vi "Climbing2.vi"(0 "Start":bool) -> ()   [LabVIEW 2018]
uses:
  <vilib>/Rock Robotics/WPI/Solenoid/WPI_SolenoidValue.ctl
  <vilib>/Rock Robotics/WPI/Utilities/WPI_GetSetVariantRefNum.vi
  Robot Global Data.vi
  <vilib>/Rock Robotics/WPI/Solenoid/WPI_SolenoidSetEnum.vi
  <vilib>/Rock Robotics/WPI/RobotDrive/WPI_RobotDriveArcadeDrive_Standard(NoSaturation).vi
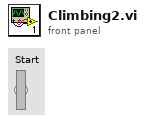
[diagram p1: front panel]
types:
  T1 = typedef "WPI_DigitalInputDevRef.ctl" = cluster{"DevStatus":errorcluster, "DIO Channel":T2}
  T2 = typedef "FPGA_DIOChannel.ctl" = enum8{"DIO 0", "DIO 1", "DIO 2", "DIO 3", "DIO 4", "DIO 5", "DIO 6", "DIO 7", "DIO 8", "DIO 9", "DIO MXP 0", "DIO MXP 1", "DIO MXP 2", "DIO MXP 3", "DIO MXP 4", "DIO MXP 5", "DIO MXP 6", "DIO MXP 7", "DIO MXP 8", "DIO MXP 9", "DIO MXP 10", "DIO MXP 11", "DIO MXP 12", "DIO MXP 13", "DIO MXP 14", "DIO MXP 15", "SPI Port CS1", "SPI Port CS2", "SPI Port CS3", "SPI Port MISO", "SPI Port MOSI", "Invalid"}
  T3 = typedef "WPI_SolenoidDevRef.ctl" = cluster{"DevStatus":errorcluster, "Pneumatics Control Module":u8, "Forward Solenoid Channel":T4, "Reverse Solenoid Channel":T4}
  T4 = typedef "WPI_SolenoidChannel.ctl" = enum8{"Solenoid 0", "Solenoid 1", "Solenoid 2", "Solenoid 3", "Solenoid 4", "Solenoid 5", "Solenoid 6", "Solenoid 7", "Invalid"}
  T5 = typedef "WPI_RobotDriveDevRef.ctl" = cluster{"DevStatus":errorcluster, "Motors[]":T6[], "Square Inputs":bool, "Max Output":dbl}
  T6 = typedef "WPI_MotorControlDeviceRef.ctl" = cluster{"DeviceStatus":errorcluster, "Type":T7, "PWM":cluster{"PWM Channel":T8, "DeadBand":T9}, "CAN":cluster{"Device Number":u8, "SetOutput VI Ref":variant, "GetOutput VI Ref":variant, "Enable VI Ref":variant, "Disable VI Ref":variant, "Data":variant}, "Invert":bool, "DIO PWM":cluster{"PWM \"Enable\" Channel":T8, "DIOChannel":T2, "PWM Rate":dbl}}
  T7 = typedef "WPI_MotorControlType.ctl" = enum16{"PWM", "CAN", "DIO PWM"}
  T8 = typedef "FPGA_DIOPWMChannel.ctl" = enum8{"PWM 0", "PWM 1", "PWM 2", "PWM 3", "PWM 4", "PWM 5", "PWM 6", "PWM 7", "PWM 8", "PWM 9", "PWM MXP 0", "PWM MXP 1", "PWM MXP 2", "PWM MXP 3", "PWM MXP 4", "PWM MXP 5", "PWM MXP 6", "PWM MXP 7", "PWM MXP 8", "PWM MXP 9", "Invalid"}
  T9 = typedef "WPI_PWMDeadband.ctl" = cluster{"Name":string, "maxPositivePwm":i32, "minPositivePwm":i32, "centerPwm":i32, "maxNegativePwm":i32, "minNegativePwm":i32, "angularRange":u16}
  T10 = typedef "WPI_SolenoidValue.ctl" = enum16{"Off", "On", "Forward", "Reverse"}
  T11 = cluster{"X-Axis":dbl, "Y-Axis":dbl, "Z-Axis":dbl}
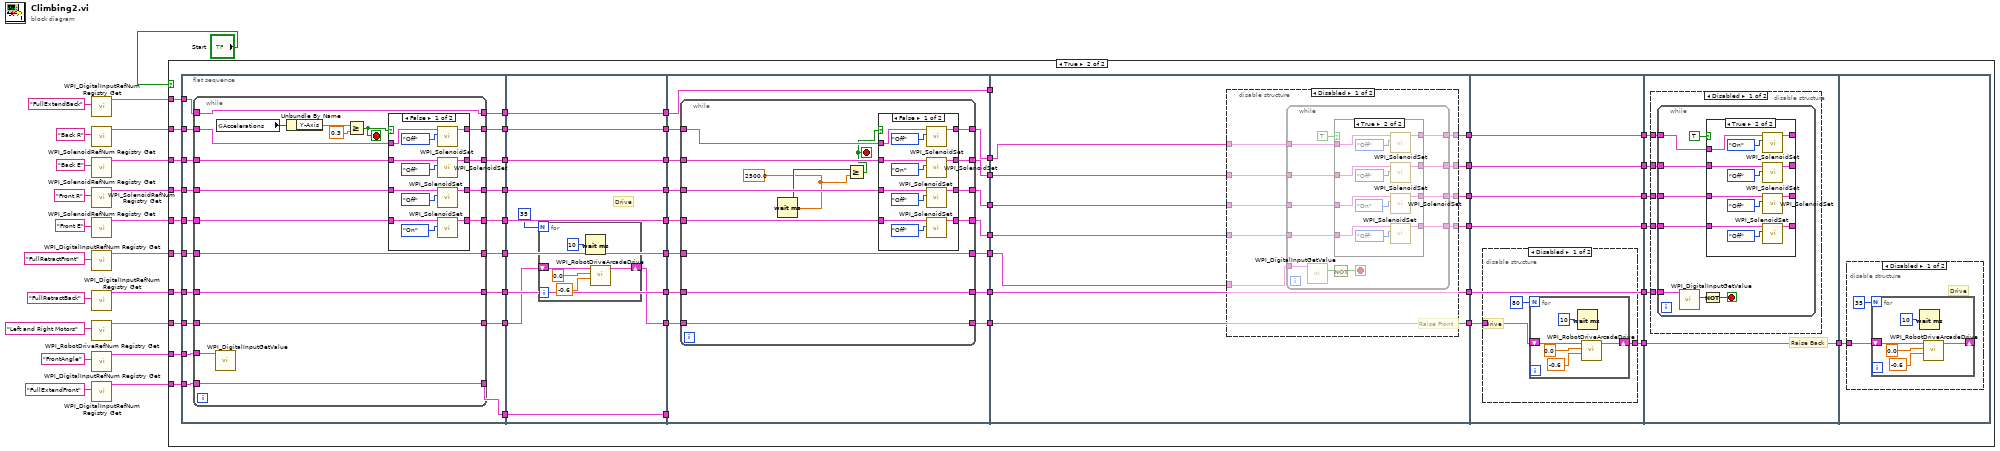
[diagram p0: block diagram]
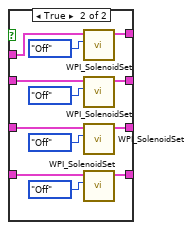
[diagram p3: hidden frame]
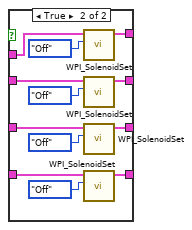
[diagram p4: hidden frame]
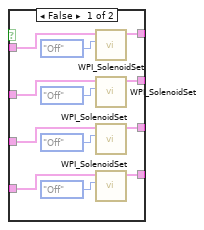
[diagram p5: hidden frame]
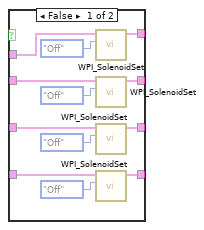
[diagram p8: hidden frame]
diagram:
  n1 = call <vilib>:"WPI_DigitalInputRefNum Registry Get.vi"("refnum name"="FullExtendBack") -> ("DigitalInputDevRef"=w21:T1)  [unwired: 9 in, 1 out]
  n2 = call <vilib>:"WPI_SolenoidRefNum Registry Get.vi"("refnum name"="Back R") -> ("SolenoidDevRef"=w9:T3)  [unwired: 9 in, 1 out]
  n3 = call <vilib>:"WPI_SolenoidRefNum Registry Get.vi"("refnum name"="Back E") -> ("SolenoidDevRef"=w7:T3)  [unwired: 9 in, 1 out]
  n4 = call <vilib>:"WPI_SolenoidRefNum Registry Get.vi"("refnum name"="Front R") -> ("SolenoidDevRef"=w8:T3)  [unwired: 9 in, 1 out]
  n5 = call <vilib>:"WPI_SolenoidRefNum Registry Get.vi"("refnum name"="Front E") -> ("SolenoidDevRef"=w6:T3)  [unwired: 9 in, 1 out]
  n6 = call <vilib>:"WPI_DigitalInputRefNum Registry Get.vi"("refnum name"="FullRetractFront") -> ("DigitalInputDevRef"=w19:T1)  [unwired: 9 in, 1 out]
  n7 = call <vilib>:"WPI_DigitalInputRefNum Registry Get.vi"("refnum name"="FullRetractBack") -> ("DigitalInputDevRef"=w17:T1)  [unwired: 9 in, 1 out]
  n8 = call <vilib>:"WPI_RobotDriveRefNum Registry Get.vi"("refnum name"="Left and Right Motors") -> ("RobotDriveDevRef"=w11:T5)  [unwired: 9 in, 1 out]
  n9 = call <vilib>:"WPI_DigitalInputRefNum Registry Get.vi"("refnum name"="FrontAngle") -> ("DigitalInputDevRef"=w15:T1)  [unwired: 9 in, 1 out]
  n10 = call <vilib>:"WPI_DigitalInputRefNum Registry Get.vi"("refnum name"="FullExtendFront") -> ("DigitalInputDevRef"=w13:T1)  [unwired: 9 in, 1 out]
  n11 = case shown="True" "Start" {
    tunnel: w6 -> [_ w70]
    tunnel: w7 -> [_ w68]
    tunnel: w8 -> [_ w69]
    tunnel: w9 -> [_ w67]
    tunnel: w11 -> [_ w66]
    tunnel: w13 -> [_ w64]
    tunnel: w15 -> [_ w65]
    tunnel: w17 -> [_ w61]
    tunnel: w19 -> [_ w62]
    tunnel: w21 -> [_ w63]
    frame False {
    }
    frame True {
      n12 = flat-sequence {
        tunnel: w70 -> [w80]
        tunnel: w69 -> [w81]
        tunnel: w68 -> [w82]
        tunnel: w67 -> [w83]
        tunnel: w66 -> [w87]
        tunnel: w65 -> [w84]
        tunnel: w64 -> [w85]
        tunnel: w63 -> [w86]
        tunnel: w62 -> [w89]
        tunnel: w61 -> [w88]
        tunnel: [w79] -> w23
        tunnel: [w78] -> w25
        tunnel: [w77] -> w27
        tunnel: [w76] -> w29
        tunnel: [w75] -> w31
        tunnel: [w74] -> w33
        tunnel: [w73] -> w35
        tunnel: [w72] -> w37
        tunnel: [w71] -> w39
        tunnel: w39 -> [w142]
        tunnel: [w142] -> w38
        tunnel: w37 -> [w141]
        tunnel: [w141] -> w36
        tunnel: w35 -> [w140]
        tunnel: [w140] -> w34
        tunnel: w33 -> [w139]
        tunnel: [w139] -> w32
        tunnel: w31 -> [w138]
        tunnel: [w138] -> w30
        tunnel: w29 -> [w137]
        tunnel: [w137] -> w28
        tunnel: w27 -> [w133]
        tunnel: [w132] -> w26
        tunnel: w25 -> [w136]
        tunnel: [w136] -> w24
        tunnel: w23 -> [w135]
        tunnel: [w135] -> w22
        tunnel: [w162] -> w60
        tunnel: [w148] -> w59
        tunnel: [w149] -> w58
        tunnel: [w150] -> w57
        tunnel: [w151] -> w56
        tunnel: [w161] -> w55
        tunnel: [w160] -> w53
        tunnel: [w159] -> w42
        tunnel: w38 -> [w162]
        tunnel: w36 -> [_]
        tunnel: w34 -> [w152]
        tunnel: w32 -> [w153]
        tunnel: w30 -> [w154]
        tunnel: w28 -> [w155]
        tunnel: w26 -> [w156]
        tunnel: w24 -> [w157]
        tunnel: w22 -> [w158]
        tunnel: [w210] -> w54
        tunnel: [w209] -> w52
        tunnel: [w208] -> w49
        tunnel: [w207] -> w47
        tunnel: [w206] -> w45
        tunnel: [w205] -> w43
        tunnel: w60 -> [_]
        tunnel: w59 -> [w201]
        tunnel: w58 -> [w202]
        tunnel: w57 -> [w203]
        tunnel: w56 -> [w204]
        tunnel: w55 -> [w211]
        tunnel: w53 -> [w210]
        tunnel: w42 -> [w205]
        tunnel: w54 -> [w263]
        tunnel: w52 -> [w262]
        tunnel: [w262] -> w51
        tunnel: [w261] -> w50
        tunnel: w49 -> [w261]
        tunnel: [w260] -> w48
        tunnel: w47 -> [w260]
        tunnel: [w259] -> w46
        tunnel: w45 -> [w259]
        tunnel: [w258] -> w44
        tunnel: w43 -> [w258]
        tunnel: [w257] -> w40
        tunnel: w51 -> [w277]
        tunnel: w50 -> [w276]
        tunnel: w48 -> [w275]
        tunnel: w46 -> [w274]
        tunnel: w44 -> [w273]
        tunnel: [w272] -> w41
        tunnel: w40 -> [w272]
        tunnel: w41 -> [w315]
        frame #0 {
          n13 = while {
            tunnel: w80 -> [w107]
            tunnel: w81 -> [w106]
            tunnel: w82 -> [w105]
            tunnel: w83 -> [w104]
            tunnel: [w103] -> w74
            tunnel: [w102] -> w73
            tunnel: [w101] -> w75
            tunnel: [w100] -> w76
            tunnel: [w99] -> w77
            tunnel: w87 -> [w99]
            tunnel: w84 -> [w98]
            tunnel: [w97] -> w72
            tunnel: w85 -> [w97]
            tunnel: [w96] -> w71
            tunnel: w86 -> [w96]
            tunnel: [w95] -> w79
            tunnel: w89 -> [w95]
            tunnel: [w94] -> w78
            tunnel: w88 -> [w94]
            stop <- w90 stop-if-true
            n14 = call <vilib>:"WPI_DigitalInputGetValue.vi"("DigitalInputDevRef"=w98) -> ()  [unwired: 8 in, 3 out]
            n15 = global read "Robot Global Data.vi" "Accelerations"() -> (w93:T11)
            n16 = Unbundle By Name(w93) -> ("Y-Axis"=w92:dbl)
            n17 = Greater Or Equal?(x=w92, y=0.3) -> (x >= y?=w90:bool)
            n18 = case shown="False" w90 {
              tunnel: w107 -> [w115 w124]
              tunnel: w106 -> [w114 w125]
              tunnel: w105 -> [w113 w126]
              tunnel: w104 -> [w112 w127]
              tunnel: [w111 w120] -> w102
              tunnel: [w110 w121] -> w103
              tunnel: [w109 w122] -> w101
              tunnel: [w108 w123] -> w100
              frame False {
                n19 = call-poly <vilib>:"WPI_SolenoidSet.vi"("Value"=WPI_SolenoidValue."Off", "SolenoidDevRef"=w112) -> ("SolenoidDevRef"=w108:T3)  [unwired: 8 in, 1 out]
                n20 = call-poly <vilib>:"WPI_SolenoidSet.vi"("Value"=WPI_SolenoidValue."Off", "SolenoidDevRef"=w113) -> ("SolenoidDevRef"=w109:T3)  [unwired: 8 in, 1 out]
                n21 = call-poly <vilib>:"WPI_SolenoidSet.vi"("Value"=WPI_SolenoidValue."Off", "SolenoidDevRef"=w114) -> ("SolenoidDevRef"=w110:T3)  [unwired: 8 in, 1 out]
                n22 = call-poly <vilib>:"WPI_SolenoidSet.vi"("Value"=WPI_SolenoidValue."On", "SolenoidDevRef"=w115) -> ("SolenoidDevRef"=w111:T3)  [unwired: 8 in, 1 out]
              }
              frame True {
                n23 = call-poly <vilib>:"WPI_SolenoidSet.vi"("Value"=WPI_SolenoidValue."Off", "SolenoidDevRef"=w127) -> ("SolenoidDevRef"=w123:T3)  [unwired: 8 in, 1 out]
                n24 = call-poly <vilib>:"WPI_SolenoidSet.vi"("Value"=WPI_SolenoidValue."Off", "SolenoidDevRef"=w126) -> ("SolenoidDevRef"=w122:T3)  [unwired: 8 in, 1 out]
                n25 = call-poly <vilib>:"WPI_SolenoidSet.vi"("Value"=WPI_SolenoidValue."Off", "SolenoidDevRef"=w125) -> ("SolenoidDevRef"=w121:T3)  [unwired: 8 in, 1 out]
                n26 = call-poly <vilib>:"WPI_SolenoidSet.vi"("Value"=WPI_SolenoidValue."Off", "SolenoidDevRef"=w124) -> ("SolenoidDevRef"=w120:T3)  [unwired: 8 in, 1 out]
              }
            }
          }
        }
        frame #1 {
          # "Drive"
          n27 = for {
            N: 35 -> [_]
            shift-right: [w147] -> w132
            shift-left: w133 -> [w146]
            n28 = Wait (ms)(milliseconds to wait=u32 10) -> ()  [unwired: 1 out]
            n29 = call-poly <vilib>:"WPI_RobotDriveArcadeDrive.vi"("Y axis value"=-0.6, "X axis value"=0.0, "RobotDriveDevRef"=w146) -> ("RobotDriveDevRef"=w147:T5)  [unwired: 6 in, 2 out]
          }
        }
        frame #2 {
          n30 = while {
            tunnel: w155 -> [w176]
            tunnel: w154 -> [w175]
            tunnel: w153 -> [w174]
            tunnel: w152 -> [w173]
            tunnel: [w172] -> w160
            tunnel: w156 -> [w172]
            tunnel: [w171] -> w151
            tunnel: [w170] -> w150
            tunnel: [w169] -> w149
            tunnel: [w168] -> w148
            tunnel: [w167] -> w161
            tunnel: w158 -> [w167]
            tunnel: [w166] -> w159
            tunnel: w157 -> [w166]
            stop <- w163 stop-if-true
            w164 = 2500.0
            n31 = Wait (ms)(milliseconds to wait=w164) -> (millisecond timer value=w165:u32)
            n32 = Greater Or Equal?(x=w165, y=w164) -> (x >= y?=w163:bool)
            n33 = case shown="False" w163 {
              tunnel: w173 -> [w184 w193]
              tunnel: w174 -> [w183 w194]
              tunnel: w175 -> [w182 w195]
              tunnel: w176 -> [w181 w196]
              tunnel: [w180 w192] -> w168
              tunnel: [w179 w191] -> w169
              tunnel: [w178 w190] -> w170
              tunnel: [w177 w189] -> w171
              frame False {
                n34 = call-poly <vilib>:"WPI_SolenoidSet.vi"("Value"=WPI_SolenoidValue."Off", "SolenoidDevRef"=w181) -> ("SolenoidDevRef"=w177:T3)  [unwired: 8 in, 1 out]
                n35 = call-poly <vilib>:"WPI_SolenoidSet.vi"("Value"=WPI_SolenoidValue."On", "SolenoidDevRef"=w182) -> ("SolenoidDevRef"=w178:T3)  [unwired: 8 in, 1 out]
                n36 = call-poly <vilib>:"WPI_SolenoidSet.vi"("Value"=WPI_SolenoidValue."Off", "SolenoidDevRef"=w183) -> ("SolenoidDevRef"=w179:T3)  [unwired: 8 in, 1 out]
                n37 = call-poly <vilib>:"WPI_SolenoidSet.vi"("Value"=WPI_SolenoidValue."Off", "SolenoidDevRef"=w184) -> ("SolenoidDevRef"=w180:T3)  [unwired: 8 in, 1 out]
              }
              frame True {
                n38 = call-poly <vilib>:"WPI_SolenoidSet.vi"("Value"=WPI_SolenoidValue."Off", "SolenoidDevRef"=w196) -> ("SolenoidDevRef"=w189:T3)  [unwired: 8 in, 1 out]
                n39 = call-poly <vilib>:"WPI_SolenoidSet.vi"("Value"=WPI_SolenoidValue."Off", "SolenoidDevRef"=w195) -> ("SolenoidDevRef"=w190:T3)  [unwired: 8 in, 1 out]
                n40 = call-poly <vilib>:"WPI_SolenoidSet.vi"("Value"=WPI_SolenoidValue."Off", "SolenoidDevRef"=w194) -> ("SolenoidDevRef"=w191:T3)  [unwired: 8 in, 1 out]
                n41 = call-poly <vilib>:"WPI_SolenoidSet.vi"("Value"=WPI_SolenoidValue."Off", "SolenoidDevRef"=w193) -> ("SolenoidDevRef"=w192:T3)  [unwired: 8 in, 1 out]
              }
            }
          }
        }
        frame #3 {
          n42 = disable-structure shown="Disabled" {
            disable-tunnel: w211 -> [w220 _]
            disable-tunnel: [w219 _] -> w209
            disable-tunnel: [w218 _] -> w208
            disable-tunnel: [w217 _] -> w207
            disable-tunnel: [w216 _] -> w206
            disable-tunnel: w204 -> [w215 _]
            disable-tunnel: w203 -> [w214 _]
            disable-tunnel: w202 -> [w213 _]
            disable-tunnel: w201 -> [w212 _]
            frame Disabled {
              # "Raise Front"
              n43 = while {
                tunnel: w220 -> [w232]
                tunnel: w212 -> [w228]
                tunnel: w213 -> [w227]
                tunnel: w214 -> [w226]
                tunnel: w215 -> [w225]
                tunnel: [w224] -> w219
                tunnel: [w223] -> w218
                tunnel: [w222] -> w217
                tunnel: [w221] -> w216
                stop <- w230 stop-if-true
                n44 = call <vilib>:"WPI_DigitalInputGetValue.vi"("DigitalInputDevRef"=w232) -> ("Value"=w231:bool)  [unwired: 8 in, 2 out]
                n45 = Not(x=w231) -> (.not. x?=w230:bool)
                n46 = case shown="True" TRUE {
                  tunnel: w228 -> [w240 w249]
                  tunnel: w227 -> [w239 w250]
                  tunnel: w226 -> [w238 w251]
                  tunnel: w225 -> [w237 w252]
                  tunnel: [w236 w248] -> w224
                  tunnel: [w235 w247] -> w223
                  tunnel: [w234 w246] -> w222
                  tunnel: [w233 w245] -> w221
                  frame False {
                    n47 = call-poly <vilib>:"WPI_SolenoidSet.vi"("Value"=WPI_SolenoidValue."Off", "SolenoidDevRef"=w237) -> ("SolenoidDevRef"=w233:T3)  [unwired: 8 in, 1 out]
                    n48 = call-poly <vilib>:"WPI_SolenoidSet.vi"("Value"=WPI_SolenoidValue."Off", "SolenoidDevRef"=w238) -> ("SolenoidDevRef"=w234:T3)  [unwired: 8 in, 1 out]
                    n49 = call-poly <vilib>:"WPI_SolenoidSet.vi"("Value"=WPI_SolenoidValue."Off", "SolenoidDevRef"=w239) -> ("SolenoidDevRef"=w235:T3)  [unwired: 8 in, 1 out]
                    n50 = call-poly <vilib>:"WPI_SolenoidSet.vi"("Value"=WPI_SolenoidValue."Off", "SolenoidDevRef"=w240) -> ("SolenoidDevRef"=w236:T3)  [unwired: 8 in, 1 out]
                  }
                  frame True {
                    n51 = call-poly <vilib>:"WPI_SolenoidSet.vi"("Value"=WPI_SolenoidValue."Off", "SolenoidDevRef"=w252) -> ("SolenoidDevRef"=w245:T3)  [unwired: 8 in, 1 out]
                    n52 = call-poly <vilib>:"WPI_SolenoidSet.vi"("Value"=WPI_SolenoidValue."Off", "SolenoidDevRef"=w251) -> ("SolenoidDevRef"=w246:T3)  [unwired: 8 in, 1 out]
                    n53 = call-poly <vilib>:"WPI_SolenoidSet.vi"("Value"=WPI_SolenoidValue."On", "SolenoidDevRef"=w250) -> ("SolenoidDevRef"=w247:T3)  [unwired: 8 in, 1 out]
                    n54 = call-poly <vilib>:"WPI_SolenoidSet.vi"("Value"=WPI_SolenoidValue."Off", "SolenoidDevRef"=w249) -> ("SolenoidDevRef"=w248:T3)  [unwired: 8 in, 1 out]
                  }
                }
              }
            }
            frame Enabled {
            }
          }
        }
        frame #4 {
          n55 = disable-structure shown="Disabled" {
            disable-tunnel: w263 -> [w265 _]
            disable-tunnel: [w264 _] -> w257
            frame Disabled {
              # "Drive"
              n56 = for {
                N: 80 -> [_]
                shift-right: [w271] -> w264
                shift-left: w265 -> [w270]
                n57 = Wait (ms)(milliseconds to wait=u32 10) -> ()  [unwired: 1 out]
                n58 = call-poly <vilib>:"WPI_RobotDriveArcadeDrive.vi"("Y axis value"=-0.6, "X axis value"=0.0, "RobotDriveDevRef"=w270) -> ("RobotDriveDevRef"=w271:T5)  [unwired: 6 in, 2 out]
              }
            }
            frame Enabled {
            }
          }
        }
        frame #5 {
          # "Raise Back"
          n59 = disable-structure shown="Disabled" {
            disable-tunnel: w277 -> [w282 _]
            disable-tunnel: w276 -> [w281 _]
            disable-tunnel: w275 -> [w280 _]
            disable-tunnel: w274 -> [w279 _]
            disable-tunnel: w273 -> [w278 _]
            frame Disabled {
              n60 = while {
                tunnel: w282 -> [w287]
                tunnel: w281 -> [w286]
                tunnel: w280 -> [w285]
                tunnel: w279 -> [w284]
                tunnel: w278 -> [w283]
                stop <- w289 stop-if-true
                n61 = call <vilib>:"WPI_DigitalInputGetValue.vi"("DigitalInputDevRef"=w283) -> ("Value"=w290:bool)  [unwired: 8 in, 2 out]
                n62 = Not(x=w290) -> (.not. x?=w289:bool)
                n63 = case shown="True" TRUE {
                  tunnel: w287 -> [w298 w307]
                  tunnel: w286 -> [w297 w308]
                  tunnel: w285 -> [w296 w309]
                  tunnel: w284 -> [w295 w310]
                  tunnel: [w294 w306] -> _
                  tunnel: [w293 w305] -> _
                  tunnel: [w292 w304] -> _
                  tunnel: [w291 w303] -> _
                  frame False {
                    n64 = call-poly <vilib>:"WPI_SolenoidSet.vi"("Value"=WPI_SolenoidValue."Off", "SolenoidDevRef"=w295) -> ("SolenoidDevRef"=w291:T3)  [unwired: 8 in, 1 out]
                    n65 = call-poly <vilib>:"WPI_SolenoidSet.vi"("Value"=WPI_SolenoidValue."Off", "SolenoidDevRef"=w296) -> ("SolenoidDevRef"=w292:T3)  [unwired: 8 in, 1 out]
                    n66 = call-poly <vilib>:"WPI_SolenoidSet.vi"("Value"=WPI_SolenoidValue."Off", "SolenoidDevRef"=w297) -> ("SolenoidDevRef"=w293:T3)  [unwired: 8 in, 1 out]
                    n67 = call-poly <vilib>:"WPI_SolenoidSet.vi"("Value"=WPI_SolenoidValue."Off", "SolenoidDevRef"=w298) -> ("SolenoidDevRef"=w294:T3)  [unwired: 8 in, 1 out]
                  }
                  frame True {
                    n68 = call-poly <vilib>:"WPI_SolenoidSet.vi"("Value"=WPI_SolenoidValue."On", "SolenoidDevRef"=w310) -> ("SolenoidDevRef"=w303:T3)  [unwired: 8 in, 1 out]
                    n69 = call-poly <vilib>:"WPI_SolenoidSet.vi"("Value"=WPI_SolenoidValue."Off", "SolenoidDevRef"=w309) -> ("SolenoidDevRef"=w304:T3)  [unwired: 8 in, 1 out]
                    n70 = call-poly <vilib>:"WPI_SolenoidSet.vi"("Value"=WPI_SolenoidValue."Off", "SolenoidDevRef"=w308) -> ("SolenoidDevRef"=w305:T3)  [unwired: 8 in, 1 out]
                    n71 = call-poly <vilib>:"WPI_SolenoidSet.vi"("Value"=WPI_SolenoidValue."Off", "SolenoidDevRef"=w307) -> ("SolenoidDevRef"=w306:T3)  [unwired: 8 in, 1 out]
                  }
                }
              }
            }
            frame Enabled {
            }
          }
        }
        frame #6 {
          n72 = disable-structure shown="Disabled" {
            disable-tunnel: w315 -> [w316 _]
            frame Disabled {
              # "Drive"
              n73 = for {
                N: 35 -> [_]
                shift-right: [w322] -> _
                shift-left: w316 -> [w321]
                n74 = Wait (ms)(milliseconds to wait=u32 10) -> ()  [unwired: 1 out]
                n75 = call-poly <vilib>:"WPI_RobotDriveArcadeDrive.vi"("Y axis value"=-0.6, "X axis value"=0.0, "RobotDriveDevRef"=w321) -> ("RobotDriveDevRef"=w322:T5)  [unwired: 6 in, 2 out]
              }
            }
            frame Enabled {
            }
          }
        }
      }
    }
  }
